vi "Data_Four Gaussian.vi"(6 "seed":i32=-1, 10 "noise amplitude":dbl=0.5, 11 "# of points":i32=4000) -> (1 "Classes":i32[](array[numeric]), 3 "Data":dbl[][](array[numeric]))   [LabVIEW 2020]
uses:
  <vilib>/Analysis/NI_AALBase.lvlib
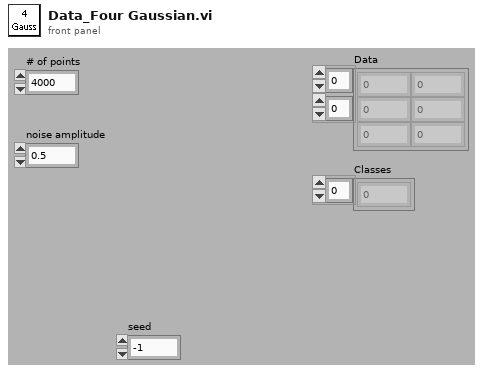
[diagram p1: front panel]
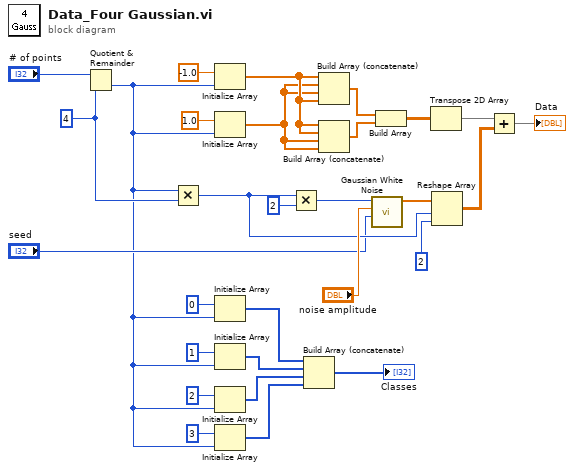
[diagram p0: block diagram]
diagram:
  w16 = 4 ("y")
  n1 = Quotient & Remainder(x="# of points", y=w16) -> (floor(x/y)=w6:i32)  [unwired: 1 out]
  n2 = Multiply(x=w6, y=w16) -> (x*y=w13:i32)
  n3 = Initialize Array(-1.0 ("element"), w6) -> (w25:dbl[])
  n4 = Initialize Array(1.0 ("element"), w6) -> (w24:dbl[])
  n5 = Initialize Array(0 ("element"), w6) -> (w5:i32[])
  n6 = Initialize Array(1 ("element"), w6) -> (w4:i32[])
  n7 = Initialize Array(2 ("element"), w6) -> (w3:i32[])
  n8 = Initialize Array(3 ("element"), w6) -> (w2:i32[])
  n9 = Multiply(x=w13, y=2) -> (x*y=w15:i32)
  n10 = Build Array (concatenate)(w5, w4, w3, w2) -> (→"Classes":i32[])
  n11 = Build Array (concatenate)(w25, w24, w24, w25) -> (w22:dbl[])
  n12 = Build Array (concatenate)(w25, w25, w24, w24) -> (w23:dbl[])
  n13 = call <vilib>:"Gaussian White Noise.vi"("seed"="seed", "standard deviation"="noise amplitude", "samples"=w15) -> ("Gaussian noise pattern"=w29:dbl[])  [unwired: 7 in, 1 out]
  n14 = Build Array(w22, w23) -> (w21:dbl[][])
  n15 = Transpose 2D Array(2D array=w21) -> (transposed array=w19:dbl[][])
  n16 = Reshape Array(w29, w13, 2 ("y")) -> (w20:dbl[][])
  n17 = Add(x=w19, y=w20) -> (x+y=→"Data":dbl[][])
